vi "Get_Dispaly_Message.vi"(0 "Oven_Data":T1, 7 "Start?":bool, 11 "Error_In":errorcluster) -> (4 "Message_Display":string, 15 "Error_Out":errorcluster)   [LabVIEW 2023]
doc: "Used to get the display message in stage and time format."
uses:
  Controls/Oven_Data.ctl
  Controls/Timer_Operation_Select.ctl
  Controls/Oven_Data_Display.ctl
  Controls/Timer_Data.ctl
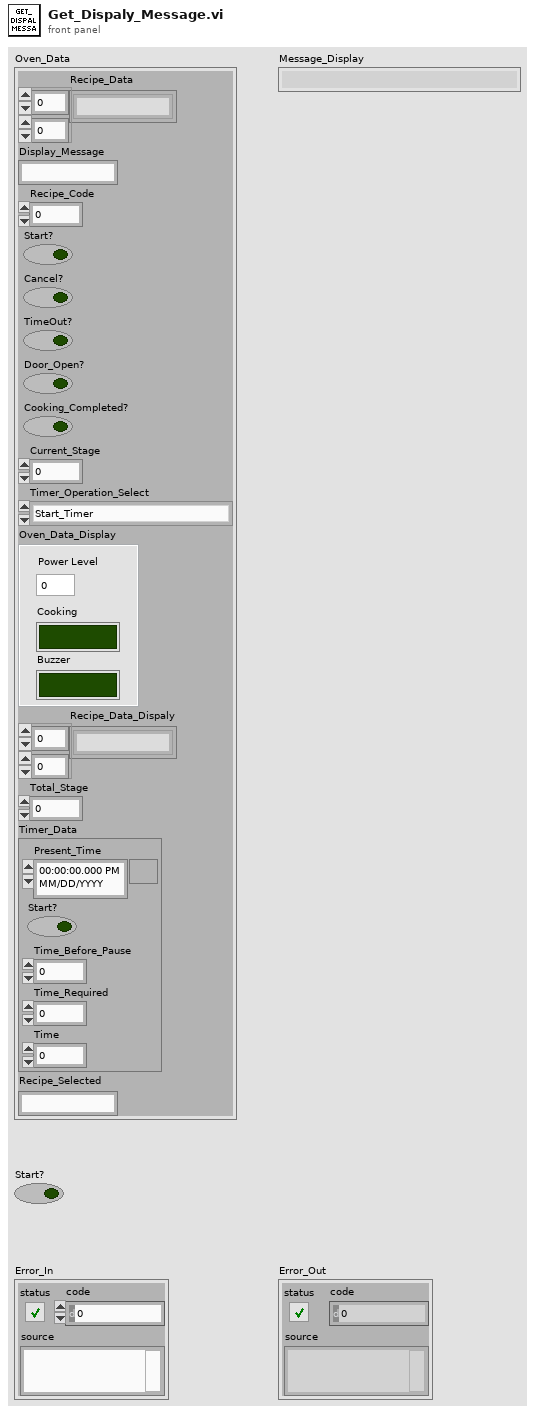
[diagram p1: front panel]
types:
  T1 = typedef "Oven_Data.ctl" = cluster{"Recipe_Data":string[][], "Display_Message":string, "Recipe_Code":i32, "Start?":bool, "Cancel?":bool, "TimeOut?":bool, "Door_Open?":bool, "Cooking_Completed?":bool, "Current_Stage":i32, "Timer_Operation_Select":T2, "Oven_Data_Display":T3, "Recipe_Data_Dispaly":string[][], "Total_Stage":i32, "Timer_Data":T4, "Recipe_Selected":string}
  T2 = typedef "Timer_Operation_Select.ctl" = enum16{"Start_Timer", "Pause_Timer", "Stop_Timer", "CheckOut_Timer"}
  T3 = typedef "Oven_Data_Display.ctl" = cluster{"Power_Level":i32, "Cooking":bool, "Buzzer":bool}
  T4 = typedef "Timer_Data.ctl" = cluster{"Present_Time":timestamp, "Start?":bool, "Time_Before_Pause":dbl, "Time_Required":dbl, "Time":dbl}
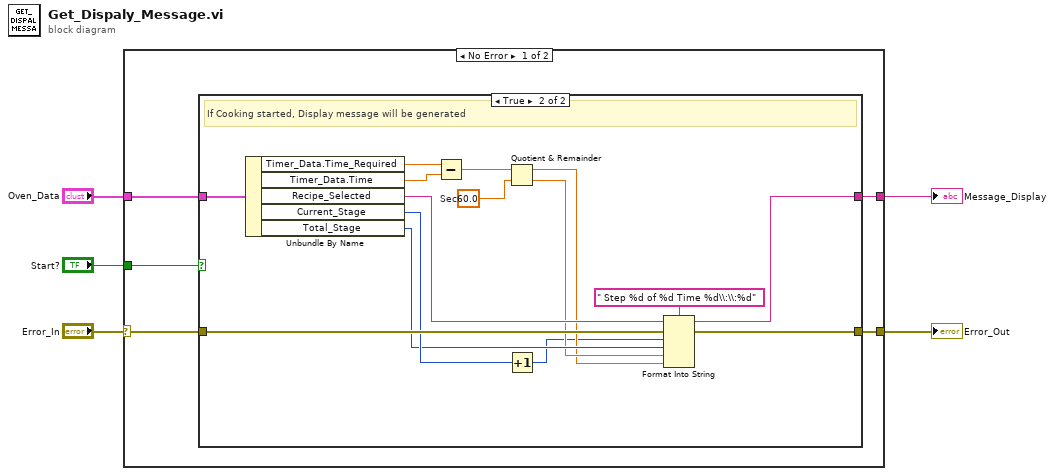
[diagram p0: block diagram]
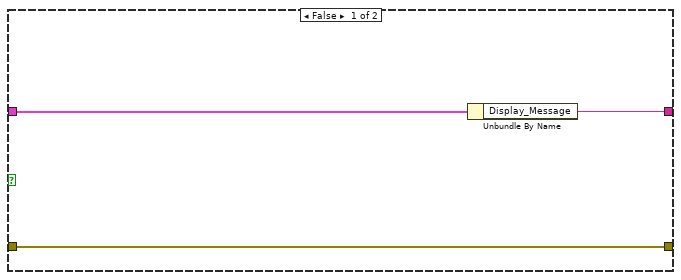
[diagram p2: hidden frame]
diagram:
  n1 = case shown="No Error" "Error_In" {
    selector: "Error_In" -> [w10 w29]
    tunnel: [w9 w29] -> w4
    tunnel: "Oven_Data" -> [w8 _]
    tunnel: [w7 _] -> w2
    tunnel: "Start?" -> [w6 _]
    frame No Error {
      n2 = case shown="True" w6 {
        tunnel: w10 -> [w13 w28]
        tunnel: [w13 w27] -> w9
        tunnel: w8 -> [w12 w23]
        tunnel: [w11 w16] -> w7
        frame False {
          n3 = Unbundle By Name(w12) -> ("Display_Message"=w11:string)
        }
        frame True {
          w24 = 60.0  # Sec
          # "If Cooking started, Display message will be generated"
          n4 = Unbundle By Name(w23) -> ("Timer_Data.Time_Required"=w25:dbl, "Timer_Data.Time"=w26:dbl, "Recipe_Selected"=w22:string, "Current_Stage"=w21:i32, "Total_Stage"=w20:i32)
          n5 = Subtract(x=w25, y=w26) -> (x-y=w15:dbl)
          n6 = Quotient & Remainder(x=w15, y=w24) -> (x-y*floor(x/y)=w18:dbl, floor(x/y)=w19:dbl)
          n7 = Increment(x=w21) -> (x+1=w14:i32)
          n8 = Format Into String(format string=" Step %d of %d Time %d\\:\\:%d", initial string=w22, error in=w28, w14, w20, w19, w18) -> (resulting string=w16:string, error out=w27:errorcluster)
        }
      }
    }
    frame Error {
    }
  }
  "Error_Out" <- w4
  "Message_Display" <- w2
